vi "FOD Y.vi"(10 "Setpoint":dbl, 11 "Setpoint":dbl) -> ()   [LabVIEW 2017]
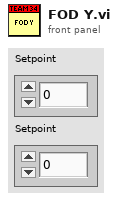
[diagram p1: front panel]
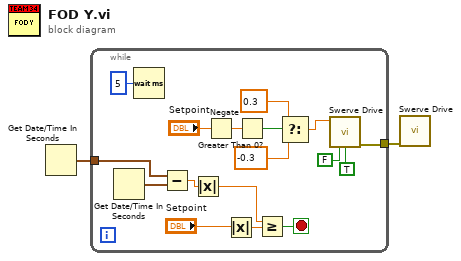
[diagram p0: block diagram]
diagram:
  n1 = Get Date/Time In Seconds() -> (seconds since 1Jan1904=w1:timestamp)
  n2 = while {
    tunnel: w1 -> [w17]
    tunnel: [w5] -> w2
    stop <- w13 stop-if-true
    n3 = Get Date/Time In Seconds() -> (seconds since 1Jan1904=w18:timestamp)
    n4 = Wait (ms)(milliseconds to wait=u32 5) -> ()  [unwired: 1 out]
    n5 = Subtract(x=w17, y=w18) -> (x-y=w16:dbl)
    n6 = Absolute Value(x=w16) -> (abs(x)=w15:dbl)
    n7 = Negate(x="Setpoint") -> (-x=w12:dbl)
    n8 = Absolute Value(x="Setpoint") -> (abs(x)=w14:dbl)
    n9 = Greater Than 0?(x=w12) -> (x > 0?=w11:bool)
    n10 = Greater Or Equal?(x=w15, y=w14) -> (x >= y?=w13:bool)
    n11 = Select(t=0.3, s=w11, f=-0.3) -> (s? t:f=w6:dbl)
    n12 = call "Swerve Drive.vi"("X"=w6, "Robot Centric?"=FALSE, "Autonomous?"=TRUE) -> ("Error Out"=w5:errorcluster)  [unwired: 8 in, 4 out]
  }
  n13 = call "Swerve Drive.vi"("Error In"=w2) -> ()  [unwired: 10 in, 5 out]
